vi "Convert Assert Event Data to Test Case - Error (APPEND) - Stack Trace is everything before Tag.vi"() -> ()   [LabVIEW 2013, in "JUnit Conversion Tests.lvlib"]
uses:
  JUnit Conversion Tests.lvlib
  <vilib>/addons/_JKI Toolkits/Caraya/classes/Test Result/Assert Event Data (Extended).ctl
  JUnit XML/Test Case/Test Case.lvclass/Test Case.ctl
  JUnit XML/Test Case/Read Stack Trace.vi
  <vilib>/addons/_JKI Toolkits/Caraya/classes/Assert/Assert Equal Value_Variant.vi
  JUnit Conversion/JUnit Conversion.lvlib
  <vilib>/addons/_JKI Toolkits/Caraya/classes/Test Result/Test Result.lvclass
  <vilib>/addons/_JKI Toolkits/Caraya/classes/Assert/Assert.lvclass
  <vilib>/addons/_JKI Toolkits/Caraya/classes/Test/Test.lvclass
  JUnit XML/Test Case/Test Case.lvclass
panel:
  out "error out":errorcluster
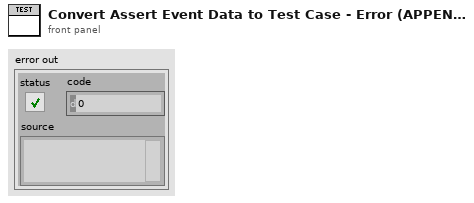
[diagram p1: front panel]
types:
  T1 = typedef "Caraya.lvlib/Test Result.lvclass/Assert Event Data (Extended).ctl" = cluster{"name":string, "passed":bool, "call-chain":string[], "test-error":errorcluster, "timestamp":timestamp, "assert-id":string, "test-id":string, "time":dbl, "message":string, "properties":variant, "measurements":variant, "user-defined":variant}
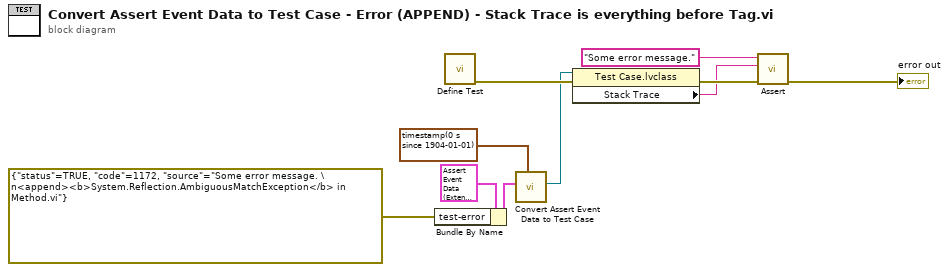
[diagram p0: block diagram]
diagram:
  n1 = Bundle By Name(cluster=T1 {"name"="", "passed"=FALSE, "call-chain"=[], "test-error"={"status"=FALSE, "code"=0, "source"=""}, "timestamp"=timestamp(0 s since 1904-01-01), "assert-id"="", "test-id"="", "time"=-1.0, "message"="", "properties"=variant, "measurements"=variant, "user-defined"=variant} ("Assert Event Data"), "test-error"=errorcluster {"status"=TRUE, "code"=1172, "source"="Some error message. \n<append><b>System.Reflection.AmbiguousMatchException</b> in Method.vi"} ("error out 2")) -> (w7:T1)
  n2 = call <vilib>:"Define Test.vi"() -> ("error out"=w9:errorcluster)  [unwired: 10 in, 1 out]
  n3 = call "Convert Assert Event Data to Test Case.vi"("Start Time"=timestamp(0 s since 1904-01-01), "Assert Event Data"=w7) -> ("Test Case"=w6:refnum<class "Test Case.lvclass">)  [unwired: 9 in]
  n4 = property class="Test Case.lvclass"(reference=w6, error in=w9) -> (error out=w5:errorcluster, "Stack Trace"=w4:string)  [unwired: 1 out]
  n5 = call-poly <vilib>:"Assert.vi"("error in (no error)"=w5, "Y"=w4, "X"="Some error message." ("message")) -> ("error out"=→"error out":errorcluster)  [unwired: 7 in, 1 out]
